vi "Stop Core.vi"(10 "final error code":i32, 11 "Camera Actor in":refnum<class "Camera Actor.lvclass">) -> (3 "Camera Actor out":refnum<class "Camera Actor.lvclass">)   [LabVIEW 2014, in "Camera Actor.lvlib" / "Camera Actor.lvclass"]
doc: "(<B>Filename</B>: Actor Framework.lvlib:Actor.lvclass:Stop Core.vi)\n\nDefines what the actor does before it stops. Use the <B>final error code</B> input to determine whether the actor shut down in response to an error.\n\nBy default, this method does nothing. A descendant class may override it to define behavior, such as shutting down any processes the actor initiated in its override of the Actor Core method."
uses:
  Camera Actor.lvclass
  Camera Actor.lvclass/Camera Actor.ctl
  <vilib>/ActorFramework/Actor/Actor.lvclass
  Logbook/Logbook/Logbook.lvclass
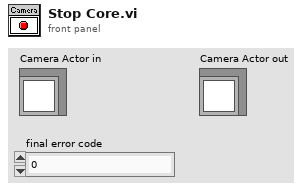
[diagram p1: front panel]
types:
  T1 = typedef "IMAQ Image.ctl" = refnum<image>
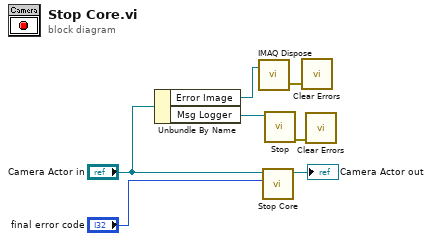
[diagram p0: block diagram]
diagram:
  n1 = Unbundle By Name("Camera Actor in") -> ("Error Image"=w2:T1, "Msg Logger"=w4:refnum<class "Logbook.lvclass">)
  n2 = call "IMAQ Dispose"("Image"=w2) -> ("error out"=w1:errorcluster)  [unwired: 5 in]
  n3 = call-parent "Stop Core.vi"("final error code"="final error code", "Actor in"="Camera Actor in") -> ("Actor out"=→"Camera Actor out":refnum<class "Camera Actor.lvclass">)  [unwired: 9 in]
  n4 = call-dynamic "Stop.vi"("Logbook in"=w4) -> ("error out"=w3:errorcluster)  [unwired: 9 in, 1 out]
  n5 = call <vilib>:"Clear Errors.vi"("error in (no error)"=w1) -> ()  [unwired: 5 in, 2 out]
  n6 = call <vilib>:"Clear Errors.vi"("error in (no error)"=w3) -> ()  [unwired: 5 in, 2 out]
